vi "Read Attributes.vi"(11 "Check Guest History Msg":refnum<class "Check Guest History Msg.lvclass">) -> (2 "Payload":cluster{"Guest Contact Number In":string})   [LabVIEW 2023, in "Guest Manager UI.lvlib" / "Check Guest History Msg.lvclass"]
uses:
  Check Guest History Msg.lvclass
  Check Guest History Msg.lvclass/Check Guest History Msg.ctl
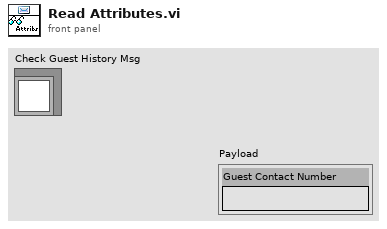
[diagram p1: front panel]
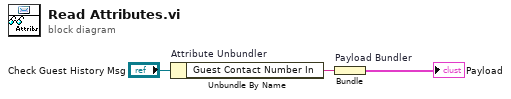
[diagram p0: block diagram]
diagram:
  n1 = Unbundle By Name "Attribute Unbundler"("Check Guest History Msg") -> ("Guest Contact Number In"=w1:string)
  n2 = Bundle "Payload Bundler"("Guest Contact Number In"=w1) -> (→"Payload":cluster{"Guest Contact Number In":string})  [unwired: 1 in]
